vi "KeyboardStringToCode.vi"(8 "error in":errorcluster, 11 "Input":T1(ring)) -> (0 "error out":errorcluster, 3 "Code":u8)   [LabVIEW 2015]
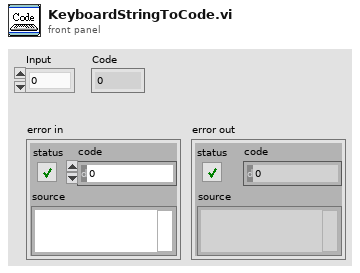
[diagram p1: front panel]
types:
  T1 = enum16{"0", "1", "2", "3", "4", "5", "6", "7", "8", "9", "A", "B", "C", "D", "E", "F", "G", "H", "I", "J", "K", "L", "M", "N", "O", "P", "Q", "R", "S", "T", "U", "V", "W", "X", "Y", "Z", "F1", "F2", "F3", "F4", "F5", "F6", "F7", "F8", "F9", "F10", "F11", "F12", "F13", "F14", "F15", "ADD", "BACK", "BACKSLASH", "CAPITAL", "COMMA", "DECIMAL", "DELETE", "DIVIDE", "DOWN", "END", "EQUALS", "ESCAPE", "GRAVE (`)", "HOME", "INSERT", "LBRACKET", "LCONTROL", "LEFT", "L ALT", "LSHIFT", "LWIN", "MINUS", "MULTIPLY", "NEXT", "NUMLOCK", "NUMPAD_0", "NUMPAD_1", "NUMPAD_2", "NUMPAD_3", "NUMPAD_4", "NUMPAD_5", "NUMPAD_6", "NUMPAD_7", "NUMPAD_8", "NUMPAD_9", "PAUSE", "PERIOD", "PRIOR (PG UP)", "RBRACKET", "RCONTROL", "RETURN", "RIGHT", "R ALT", "RSHIFT", "RWIN", "SCROLL", "SEMICOLON", "SLASH", "SPACE", "SUBTRACT", "TAB", "UP", "ENTER (num pad)", "' (quote)"}
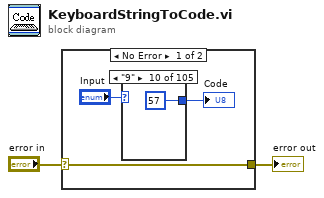
[diagram p0: block diagram]
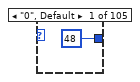
[diagram p2: hidden frame]
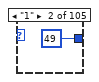
[diagram p3: hidden frame]
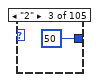
[diagram p4: hidden frame]
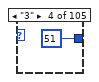
[diagram p5: hidden frame]
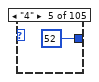
[diagram p6: hidden frame]
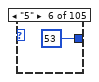
[diagram p7: hidden frame]
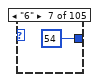
[diagram p8: hidden frame]
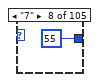
[diagram p9: hidden frame]
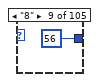
[diagram p10: hidden frame]
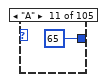
[diagram p11: hidden frame]
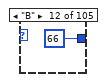
[diagram p12: hidden frame]
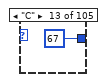
[diagram p13: hidden frame]
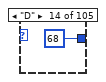
[diagram p14: hidden frame]
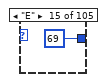
[diagram p15: hidden frame]
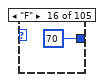
[diagram p16: hidden frame]
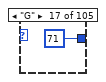
[diagram p17: hidden frame]
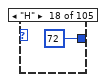
[diagram p18: hidden frame]
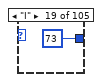
[diagram p19: hidden frame]
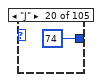
[diagram p20: hidden frame]
diagram:
  n1 = case shown="No Error" "error in" {
    selector: "error in" -> [w3 w111]
    tunnel: [w3 w111] -> w1
    frame No Error {
      n2 = case shown="\"9\"" "Input" {
        tunnel: [u8 48 u8 49 u8 50 u8 51 u8 52 u8 53 u8 54 u8 55 u8 56 u8 57 u8 65 u8 66 u8 67 u8 68 u8 69 u8 70 u8 71 u8 72 u8 73 u8 74 u8 75 u8 76 u8 77 u8 78 u8 79 u8 80 u8 81 u8 82 u8 83 u8 84 u8 85 u8 86 u8 87 u8 88 u8 89 u8 90 u8 112 u8 113 u8 114 u8 115 u8 116 u8 117 u8 118 u8 119 u8 120 u8 121 u8 122 u8 123 u8 124 u8 125 u8 126 u8 107 u8 8 u8 220 u8 20 u8 188 u8 46 u8 110 u8 111 u8 98 u8 97 u8 187 u8 27 u8 192 u8 103 u8 96 u8 219 u8 17 u8 100 u8 18 u8 16 u8 91 u8 189 u8 106 u8 99 u8 144 u8 255 u8 35 u8 40 u8 34 u8 37 u8 12 u8 39 u8 36 u8 38 u8 33 u8 144 u8 190 u8 105 u8 221 u8 163 u8 13 u8 102 u8 165 u8 161 u8 92 u8 145 u8 186 u8 191 u8 32 u8 109 u8 9 u8 104 u8 13 u8 222] -> w4
        frame "0", Default {
        }
        frame "1" {
        }
        frame "2" {
        }
        frame "3" {
        }
        frame "4" {
        }
        frame "5" {
        }
        frame "6" {
        }
        frame "7" {
        }
        frame "8" {
        }
        frame "9" {
        }
        frame "A" {
        }
        frame "B" {
        }
        frame "C" {
        }
        frame "D" {
        }
        frame "E" {
        }
        frame "F" {
        }
        frame "G" {
        }
        frame "H" {
        }
        frame "I" {
        }
        frame "J" {
        }
        frame "K" {
        }
        frame "L" {
        }
        frame "M" {
        }
        frame "N" {
        }
        frame "O" {
        }
        frame "P" {
        }
        frame "Q" {
        }
        frame "R" {
        }
        frame "S" {
        }
        frame "T" {
        }
        frame "U" {
        }
        frame "V" {
        }
        frame "W" {
        }
        frame "X" {
        }
        frame "Y" {
        }
        frame "Z" {
        }
        frame "F1" {
        }
        frame "F2" {
        }
        frame "F3" {
        }
        frame "F4" {
        }
        frame "F5" {
        }
        frame "F6" {
        }
        frame "F7" {
        }
        frame "F8" {
        }
        frame "F9" {
        }
        frame "F10" {
        }
        frame "F11" {
        }
        frame "F12" {
        }
        frame "F13" {
        }
        frame "F14" {
        }
        frame "F15" {
        }
        frame "ADD" {
        }
        frame "BACK" {
        }
        frame "BACKSLASH" {
        }
        frame "CAPITAL" {
        }
        frame "COMMA" {
        }
        frame "DECIMAL" {
        }
        frame "DELETE" {
        }
        frame "DIVIDE" {
        }
        frame "DOWN" {
        }
        frame "END" {
        }
        frame "EQUALS" {
        }
        frame "ESCAPE" {
        }
        frame "GRAVE (`)" {
        }
        frame "HOME" {
        }
        frame "INSERT" {
        }
        frame "LBRACKET" {
        }
        frame "LCONTROL" {
        }
        frame "LEFT" {
        }
        frame "L ALT" {
        }
        frame "LSHIFT" {
        }
        frame "LWIN" {
        }
        frame "MINUS" {
        }
        frame "MULTIPLY" {
        }
        frame "NEXT" {
        }
        frame "NUMLOCK" {
        }
        frame "NUMPAD_0" {
        }
        frame "NUMPAD_1" {
        }
        frame "NUMPAD_2" {
        }
        frame "NUMPAD_3" {
        }
        frame "NUMPAD_4" {
        }
        frame "NUMPAD_5" {
        }
        frame "NUMPAD_6" {
        }
        frame "NUMPAD_7" {
        }
        frame "NUMPAD_8" {
        }
        frame "NUMPAD_9" {
        }
        frame "PAUSE" {
        }
        frame "PERIOD" {
        }
        frame "PRIOR (PG UP)" {
        }
        frame "RBRACKET" {
        }
        frame "RCONTROL" {
        }
        frame "RETURN" {
        }
        frame "RIGHT" {
        }
        frame "R ALT" {
        }
        frame "RSHIFT" {
        }
        frame "RWIN" {
        }
        frame "SCROLL" {
        }
        frame "SEMICOLON" {
        }
        frame "SLASH" {
        }
        frame "SPACE" {
        }
        frame "SUBTRACT" {
        }
        frame "TAB" {
        }
        frame "UP" {
        }
        frame "ENTER (num pad)" {
        }
        frame "' (quote)" {
        }
      }
      "Code" <- w4
    }
    frame Error {
    }
  }
  "error out" <- w1
